vi "BIO_set_ssl.vi"(7 "close flag":i32=1, 8 "error in (no error)":errorcluster, 10 "SSL in":refnum<class "SSL.lvclass">, 11 "BIO in":refnum<class "BIO.lvclass">) -> (0 "error out":errorcluster, 3 "BIO out":refnum<class "BIO.lvclass">)   [LabVIEW 2013, in "SSL_Lib.lvlib" / "BIO.lvclass"]
uses:
  BIO.lvclass
  SSL/SSL.lvclass
  SSL-Lib/SSL-Lib.lvclass/SSL-Lib.ctl
  BIO.lvclass/BIO.ctl
  SSL/SSL.lvclass/SSL.ctl
  SSL/Read Handle.vi
  SSL-Lib/Read Crypto Library Path.vi
  Read Handle.vi
  SSL-Lib/SSL-Lib.lvclass
panel:
  out "return type":i32
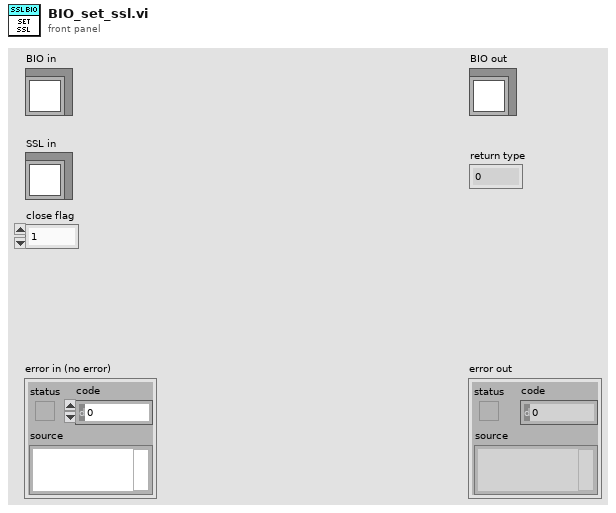
[diagram p1: front panel]
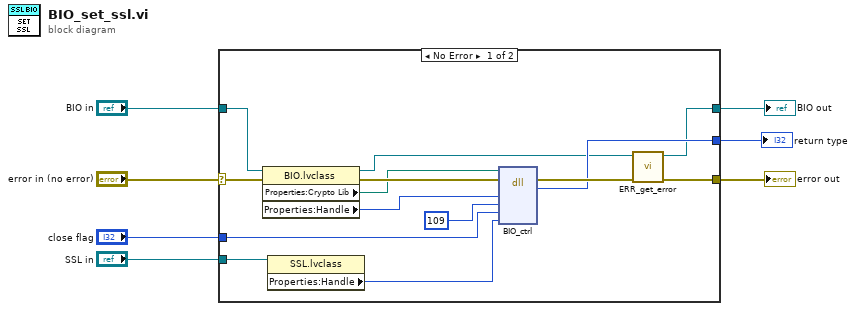
[diagram p0: block diagram]
diagram:
  n1 = case shown="No Error" "error in (no error)" {
    selector: "error in (no error)" -> [w21 w23]
    tunnel: [w12 w23] -> w6
    tunnel: [w10 w22] -> w4
    tunnel: "BIO in" -> [w15 w22]
    tunnel: [w18 _] -> w3
    tunnel: "close flag" -> [w17 _]
    tunnel: "SSL in" -> [w13 _]
    frame No Error {
      n2 = property class="BIO.lvclass"(reference=w15, error in=w21) -> (reference out=w11:refnum<class "BIO.lvclass">, error out=w16:errorcluster, "Properties:Crypto Lib"=w14:path, "Properties:Handle"=w9:u64)
      n3 = property class="SSL.lvclass"(reference=w13) -> ("Properties:Handle"=w8:u64)  [unwired: 1 in, 2 out]
      n4 = dll-call lib="C:/Program Files (x86)/National Instruments/Shared/nissl/NIssleay32.dll" fn="BIO_ctrl"(path in=w14, error in=w16, "BIO"=w9, "cmd"=109, "larg"=w17, "parg"=w8) -> (error out=w20:errorcluster, "return type"=w18:i32)  [unwired: 5 in, 1 out]
      n5 = call "ERR_get_error.vi"("error in (no error)"=w20, "SSL-Lib in"=w11) -> ("error out"=w12:errorcluster, "SSL-Lib out"=w10:refnum<class "BIO.lvclass">)  [unwired: 8 in]
    }
    frame Error {
    }
  }
  "error out" <- w6
  "BIO out" <- w4
  "return type" <- w3
